vi "Send Drive Data.vi"(1 "DVR In":refnum<data-value>) -> ()   [LabVIEW 2016]
uses:
  Drive Notifier.ctl
  Drive Control Type.ctl
  Drive Globals.vi
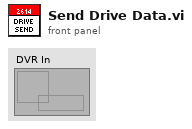
[diagram p1: front panel]
types:
  T1 = typedef "Drive Notifier.ctl" = cluster{"Parameter 1":dbl, "Parameter 2":dbl, "Parameter 3":dbl, "Drive Control List":T2, "Parameter 4":dbl, "Parameter 5":dbl, "Parameter 6":dbl, "Parameter 7":dbl, "Parameter 8":dbl, "Parameter 9":dbl}
  T2 = typedef "Drive Control Type.ctl" = enum16{"No Op", "Fieldcentric", "Robotcentric"}
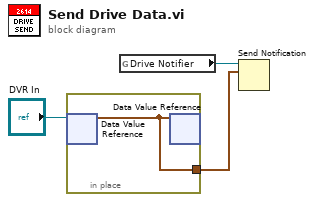
[diagram p0: block diagram]
diagram:
  n1 = in-place {
    in-place-border: [w4] -> w3
    n2 = in-place-dvr #1("DVR In") -> (w4:T1)  [unwired: 1 out]
    n3 = in-place-dvr #1(w4) -> ()  [unwired: 2 out]
  }
  n4 = global read "Drive Globals.vi" "Drive Notifier"() -> (w1:refnum<notifier>)
  n5 = Send Notification(notification=w3, notifier=w1) -> ()  [unwired: 1 in, 2 out]
